vi "run_test_item.vi"(7 "DAQmx Device Name":tag="Dev1", 8 "error in":errorcluster, 10 "Test item":T2) -> (0 "error out":errorcluster, 1 "Test result":T1, 2 "Cluster":T6 {"Time Stamp" format="%<%.3X>T"})   [LabVIEW 2019]
doc: "The VI's input is a ctl_test_item_cluster. The output is the ctl_results_cluster indicator:\n- Time stamp: is the current time\n- Test item name: is the same as the Test item control's same label\n- Efficiency, Input Voltage, Output Voltage: pass criteria fulfilment for the measurement performed (perfrom_measurement.vi) based on the Test item.Stimuli cluster, results compared to the Test item.Pass limits cluster"
uses:
  ctl_pass_fail_led.ctl
  ctl_results_cluster.ctl
  ctl_loads_enum.ctl
  ctl_stimuli_cluster.ctl
  ctl_pass_limits_cluster.ctl
  ctl_test_item_cluster.ctl
  ctl_test_outputs_cluster.ctl
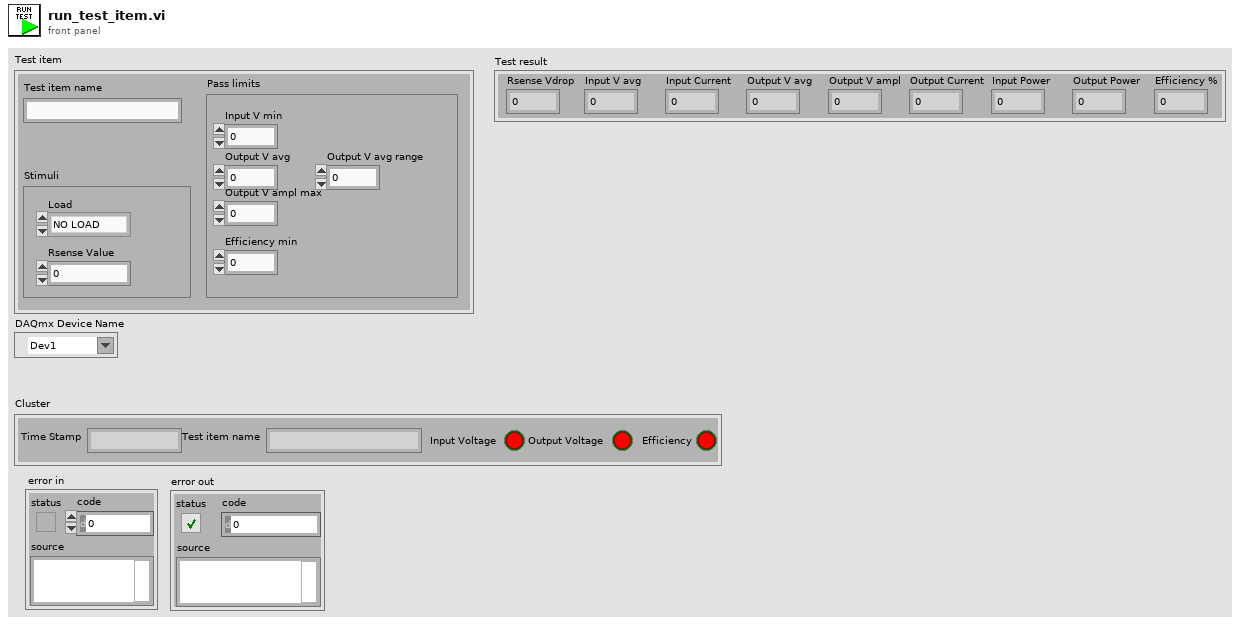
[diagram p1: front panel]
types:
  T1 = typedef "ctl_test_outputs_cluster.ctl" = cluster{"Output V avg":dbl, "Output V ampl":dbl, "Input Current":dbl, "Output Current":dbl, "Efficiency %":dbl, "Input V avg":dbl, "Input Power":dbl, "Output Power":dbl, "Rsense Vdrop":dbl}
  T2 = typedef "ctl_test_item_cluster.ctl" = cluster{"Stimuli":T3, "Pass limits":T5, "Test item name":string}
  T3 = typedef "ctl_stimuli_cluster.ctl" = cluster{"Load":T4, "Rsense Value":dbl}
  T4 = typedef "ctl_loads_enum.ctl" = enum16{"NO LOAD"}
  T5 = typedef "ctl_pass_limits_cluster.ctl" = cluster{"Output V avg":dbl, "Output V ampl max":dbl, "Efficiency min":dbl, "Input V min":dbl, "Output V avg range":dbl}
  T6 = typedef "ctl_results_cluster.ctl" = cluster{"Time Stamp":timestamp, "Test item name":string, "Input Voltage":T7, "Output Voltage":T7, "Efficiency":T7}
  T7 = typedef "ctl_pass_fail_led.ctl" = bool
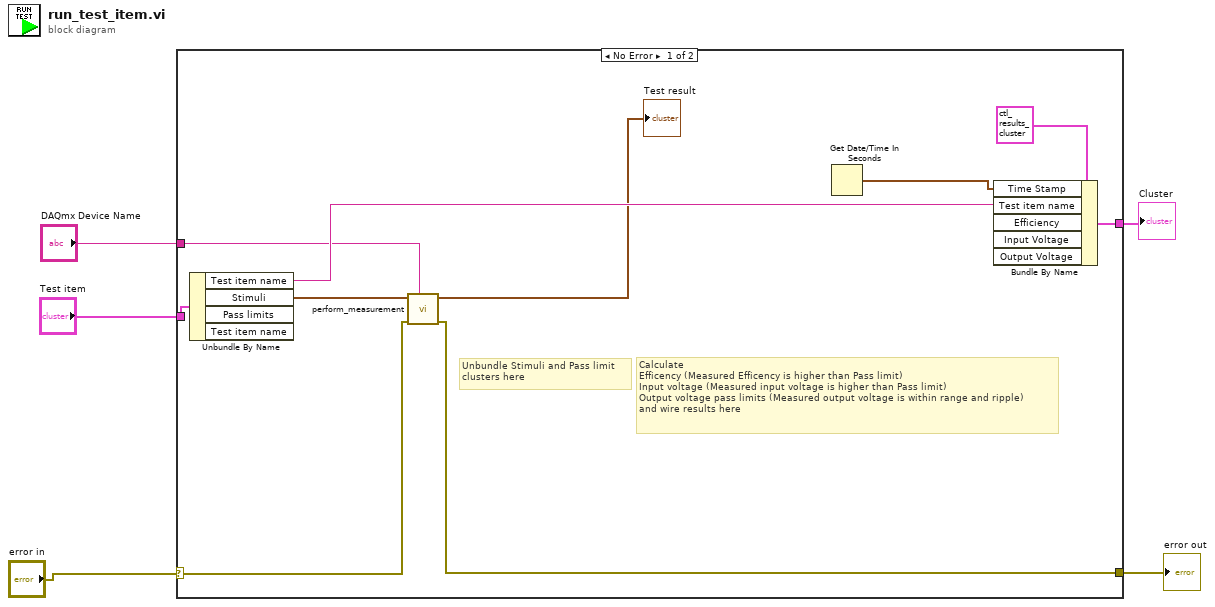
[diagram p0: block diagram]
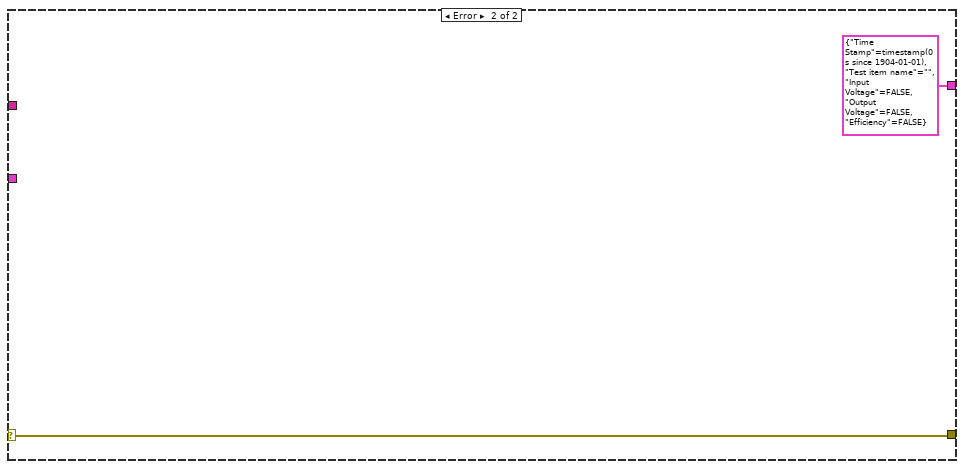
[diagram p2: hidden frame]
diagram:
  n1 = case shown="No Error" "error in" {
    selector: "error in" -> [w7 w17]
    tunnel: "Test item" -> [w15 _]
    tunnel: [w10 T6 {"Time Stamp"=timestamp(0 s since 1904-01-01), "Test item name"="", "Input Voltage"=FALSE, "Output Voltage"=FALSE, "Efficiency"=FALSE} ("Cluster")] -> w4
    tunnel: "DAQmx Device Name" -> [w9 _]
    tunnel: [w8 w17] -> w2
    frame No Error {
      # "Calculate\nEfficency (Measured Efficency is higher than Pass limit)\nInput voltage (Measured input voltage is higher than Pass limit)\nOutput voltage pass limits (Measured output voltage is within range and ripple)\nand wire results here"
      # "Unbundle Stimuli and Pass limit\nclusters here"
      n2 = Unbundle By Name(w15) -> ("Test item name"=w12:string, "Stimuli"=w14:T3)  [unwired: 2 out]
      n3 = call "perform_measurement.vi"("DAQmx Device Name"=w9, "error in"=w7, "Stimuli"=w14) -> ("error out"=w8:errorcluster, "Outputs"=→"Test result":T1)  [unwired: 6 in, 1 out]
      n4 = Get Date/Time In Seconds() -> (seconds since 1Jan1904=w11:timestamp)
      n5 = Bundle By Name(cluster=T6 {"Time Stamp"=timestamp(0 s since 1904-01-01), "Test item name"="", "Input Voltage"=FALSE, "Output Voltage"=FALSE, "Efficiency"=FALSE} ("Cluster"), "Time Stamp"=w11, "Test item name"=w12) -> (w10:T6)  [unwired: 3 in]
    }
    frame Error {
    }
  }
  "Cluster" <- w4
  "error out" <- w2
